vi "Simulation Record Get.vi"(8 "Error In":errorcluster, 11 "simulator":T20={"configuration"={"maxTime"=5.0, "enableVisualization"=TRUE, "Environment Definition"=path "iRobot Navigation State Machine.vi", "Record Location"=path "Simulation Record.xml", "autograde?"=TRUE, "interactive?"=FALSE, "Feedback Mode"=enum."debug navigation", "Robot State Charts"=[path "C:/Users/blueuser/Desktop/Robo Sim Berkley/cpsgrader-release-0.4/Simulators/EECS149lab/src/LabVIEW/statechart/Simulation Statechart.vi"], "statechart"=path "C:/Users/blueuser/Desktop/Robo Sim Berkley/cpsgrader-release-0.4/Simulators/EECS149lab/src/LabVIEW/statechart/Simulation Statechart.vi"}, "Statechart\ndisplay"=refnum, "first step?"=FALSE, "Robots Simulation Statecharts"=[], "Robots"=[]}) -> (0 "Error Out":errorcluster, 2 "record":T1={"configuration"={"maxTime"=5.0, "enableVisualization"=TRUE, "Environment Definition"=path "iRobot Navigation State Machine.vi", "Record Location"=path "Simulation Record.xml", "autograde?"=TRUE, "interactive?"=FALSE, "Feedback Mode"=enum."debug navigation", "Robot State Charts"=[path "C:/Users/blueuser/Desktop/Robo Sim Berkley/cpsgrader-release-0.4/Simulators/EECS149lab/src/LabVIEW/statechart/Simulation Statechart.vi"], "statechart"=path "C:/Users/blueuser/Desktop/Robo Sim Berkley/cpsgrader-release-0.4/Simulators/EECS149lab/src/LabVIEW/statechart/Simulation Statechart.vi"}, "trace"=[], "environment MD5"="", "statechart MD5"="", "record timestamp"=""} {"trace"."sensors"."Kobuki Sensors"."Infrared" format="%02x"; "trace"."sensors"."iRobot Sensors"."Infrared" format="%02x"; "trace"."sensors"."accelerometer"."z axis (g)" format="%.3f"; "trace"."sensors"."accelerometer"."y axis (g)" format="%.3f"; "trace"."sensors"."accelerometer"."x axis (g)" format="%.3f"}, 3 "simulator":T20={"configuration"={"maxTime"=5.0, "enableVisualization"=TRUE, "Environment Definition"=path "iRobot Navigation State Machine.vi", "Record Location"=path "Simulation Record.xml", "autograde?"=TRUE, "interactive?"=FALSE, "Feedback Mode"=enum."debug navigation", "Robot State Charts"=[path "C:/Users/blueuser/Desktop/Robo Sim Berkley/cpsgrader-release-0.4/Simulators/EECS149lab/src/LabVIEW/statechart/Simulation Statechart.vi"], "statechart"=path "C:/Users/blueuser/Desktop/Robo Sim Berkley/cpsgrader-release-0.4/Simulators/EECS149lab/src/LabVIEW/statechart/Simulation Statechart.vi"}, "Statechart\ndisplay"=refnum, "first step?"=FALSE, "Robots Simulation Statecharts"=[], "Robots"=[]})   [LabVIEW 2014]
uses:
  Simulator.ctl
  CyberSim interface/Simulation Configuration.ctl
  autograder/feedbackMode.ctl
  Multi Bot Code/RobotData.ctl
  <instrlib>/DC Motor Controller/HAIOL/DC Motor Controller.lvclass
  Simulation Record.ctl
  Simulation Trace Element.ctl
  shared/Sensors.ctl
  iRobot/Sensor/Accelerometer.ctl
  iRobot/Sensor/Sensor Group 6.ctl
  iRobot/Sensor/Bumps + Wheel Drops.ctl
  iRobot/Sensor/Buttons.ctl
  iRobot/Sensor/Charging State.ctl
  iRobot/Sensor/Charging Sources Available.ctl
  iRobot/Sensor/OI Mode.ctl
  iRobot/Sensor/Cargo Bay Digital Inputs.ctl
  iRobot/Sensor/Low-Side Driver + Wheel Overcurrent.ctl
  Kobuki/KobukiSensors.ctl
  Kobuki/Kobuki Bumps and WheelDrops.ctl
  Kobuki/Kobuki Buttons.ctl
  Simulated iRobot Position.ctl
  Simulated iRobot Orientation.ctl
  Simulation Trace Operation.ctl
panel:
  # "Electrical: charging, battery, OI mode"
  # "Sensors: bump, cliff, button, wheel drop, wall, virtual wall"
  # "Motors:"
  # "Cargo Bay: I/O, overcurrent, infrared"
  # "Song"
  # "Inertia"
  # "Electrical: charging, battery, OI mode"
  # "Sensors: bump, cliff, button, wheel drop, wall, virtual wall"
  # "Motion: distance, angle, requested velocity"
  # "Cargo Bay: I/O, overcurrent, infrared"
  # "Song"
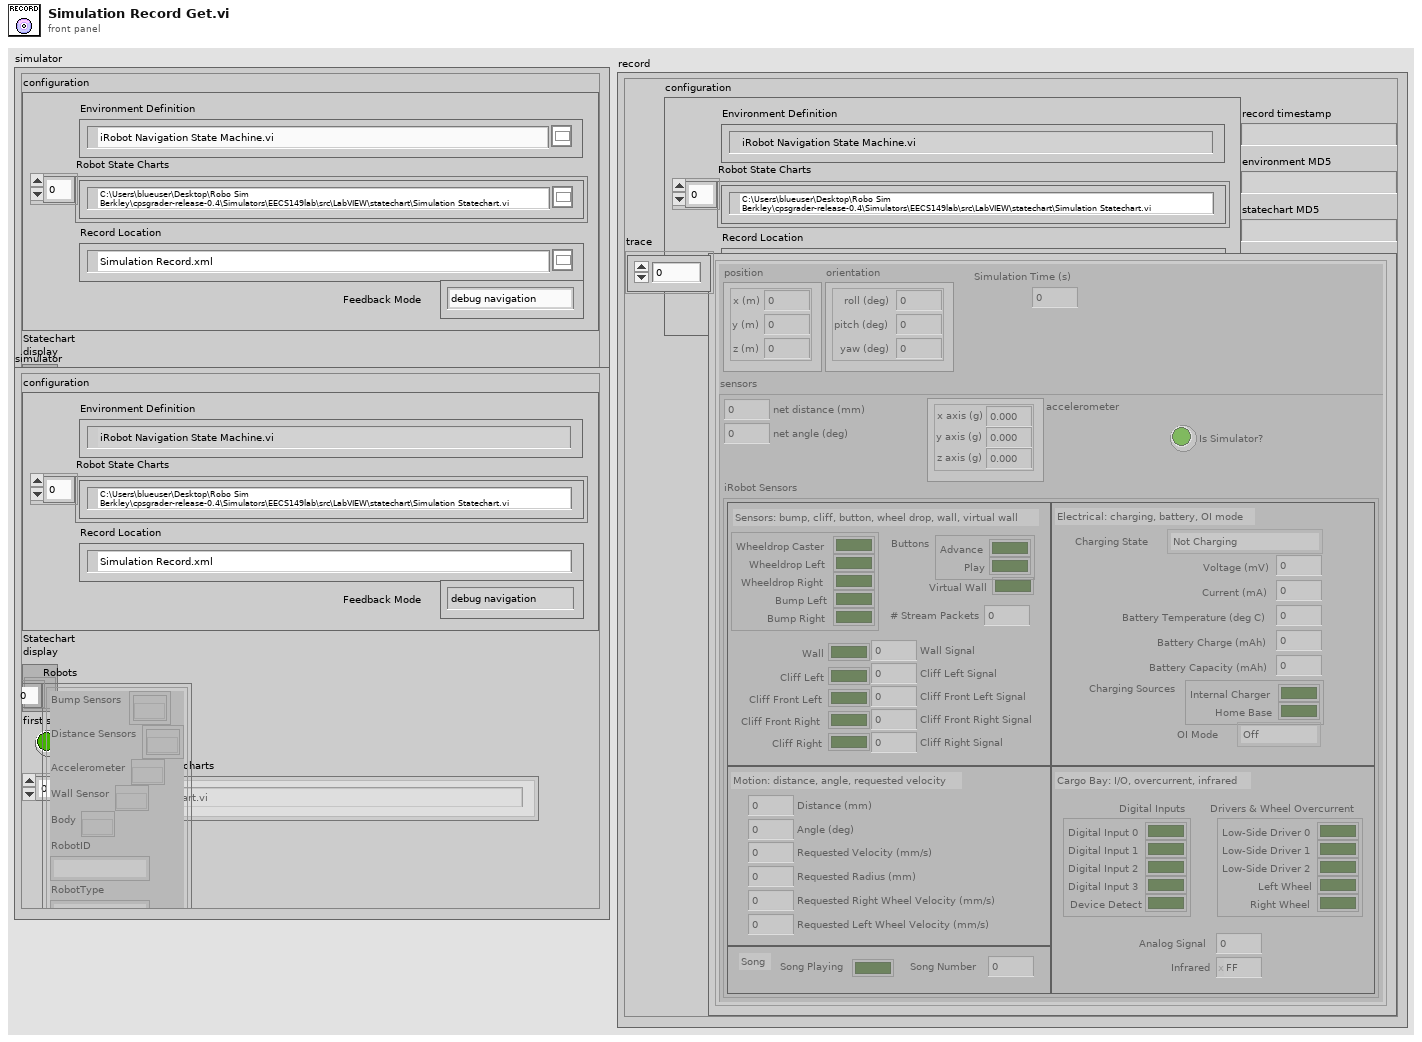
[diagram p1: front panel]
types:
  T1 = typedef "Simulation Record.ctl" = cluster{"configuration":T2, "trace":T4[], "environment MD5":string, "statechart MD5":string, "record timestamp":string}
  T2 = typedef "Simulation Configuration.ctl" = cluster{"maxTime":sgl, "enableVisualization":bool, "Environment Definition":path, "Record Location":path, "autograde?":bool, "interactive?":bool, "Feedback Mode":T3, "Robot State Charts":path[], "statechart":path}
  T3 = typedef "feedbackMode.ctl" = enum32{"debug navigation", "debug hill climb", "autograde navigation", "autograde hill climb"}
  T4 = typedef "Simulation Trace Element.ctl" = cluster{"sensors":T5, "position":T18, "orientation":T19, "Simulation Time (s)":sgl}
  T5 = typedef "Sensors.ctl" = cluster{"net distance (mm)":i32, "net angle (deg)":i32, "accelerometer":T6, "iRobot Sensors":T7, "Is Simulator?":bool, "Kobuki Sensors":T15}
  T6 = typedef "Accelerometer.ctl" = cluster{"x axis (g)":dbl, "y axis (g)":dbl, "z axis (g)":dbl}
  T7 = typedef "Sensor Group 6.ctl" = cluster{"Bumps + Wheel Drops":T8, "Wall":bool, "Cliff Left":bool, "Cliff Front Left":bool, "Cliff Front Right":bool, "Cliff Right":bool, "Wall Signal":u16, "Cliff Left Signal":u16, "Cliff Front Left Signal":u16, "Cliff Front Right Signal":u16, "Cliff Right Signal":u16, "Buttons":T9, "Virtual Wall":bool, "# Stream Packets":u8, "Requested Velocity (mm/s)":i16, "Requested Radius (mm)":i16, "Requested Right Wheel Velocity (mm/s)":i16, "Requested Left Wheel Velocity (mm/s)":i16, "Distance (mm)":i32, "Angle (deg)":i32, "Song Playing":bool, "Song Number":u8, "Charging State":T10, "Voltage (mV)":u16, "Current (mA)":i16, "Battery Temperature (deg C)":i8, "Battery Charge (mAh)":u16, "Battery Capacity (mAh)":u16, "Charging Sources":T11, "OI Mode":T12, "Digital Inputs":T13, "Drivers & Wheel Overcurrent":T14, "Analog Signal":u16, "Infrared":u8}
  T8 = typedef "Bumps + Wheel Drops.ctl" = cluster{"Wheeldrop Caster":bool, "Wheeldrop Left":bool, "Wheeldrop Right":bool, "Bump Left":bool, "Bump Right":bool}
  T9 = typedef "Buttons.ctl" = cluster{"Advance":bool, "Play":bool}
  T10 = typedef "Charging State.ctl" = enum16{"Not Charging", "Reconditioning Charging", "Full Charging", "Trickle Charging", "Waiting", "Charging Fault Condition"}
  T11 = typedef "Charging Sources Available.ctl" = cluster{"Internal Charger":bool, "Home Base":bool}
  T12 = typedef "OI Mode.ctl" = enum16{"Off", "Passive", "Safe", "Full"}
  T13 = typedef "Cargo Bay Digital Inputs.ctl" = cluster{"Digital Input 0":bool, "Digital Input 1":bool, "Digital Input 2":bool, "Digital Input 3":bool, "Device Detect":bool}
  T14 = typedef "Low-Side Driver + Wheel Overcurrent.ctl" = cluster{"Low-Side Driver 0":bool, "Low-Side Driver 1":bool, "Low-Side Driver 2":bool, "Left Wheel":bool, "Right Wheel":bool}
  T15 = typedef "KobukiSensors.ctl" = cluster{"Bumps + Wheel Drops":T16, "Cliff Left":bool, "Cliff Center":bool, "Cliff Right":bool, "Cliff Left Signal":i16, "Cliff Center Signal":i16, "Cliff Right Signal":i16, "Buttons":T17, "Left Wheel Encoder (ticks)":i16, "Song Playing":bool, "Song Number":u8, "Charging State":T10, "Voltage (mV)":i16, "Current (mA)":i16, "Battery Temperature (deg C)":i16, "Battery Charge (mAh)":i16, "Battery Capacity (mAh)":i16, "Charging Sources":T11, "OI Mode":T12, "Digital Inputs":T13, "Drivers & Wheel Overcurrent":T14, "Infrared":u8, "Right Wheel Encoder (ticks) ":i16, "TimeStamp":u16, "Right Wheel Current (x10mA)":i16, "Left  Wheel Current  (x10mA)":i16, "Angle( of 100deg)":i16, "Angle Rate( of 100 deg/sec)":i16}
  T16 = typedef "Kobuki Bumps and WheelDrops.ctl" = cluster{"Wheeldrop Left":bool, "Wheeldrop Right":bool, "Bump Left":bool, "Bump Center":bool, "Bump Right":bool}
  T17 = typedef "Kobuki Buttons.ctl" = cluster{"B0":bool, "B1":bool, "B2":bool}
  T18 = typedef "Simulated iRobot Position.ctl" = cluster{"x (m)":sgl, "y (m)":sgl, "z (m)":sgl}
  T19 = typedef "Simulated iRobot Orientation.ctl" = cluster{"roll (deg)":sgl, "pitch (deg)":sgl, "yaw (deg)":sgl}
  T20 = typedef "Simulator.ctl" = cluster{"configuration":T2, "Statechart\ndisplay":refnum<vi>, "first step?":bool, "Robots Simulation Statecharts":path[], "Robots":T21[]}
  T21 = typedef "RobotData.ctl" = cluster{"Bump Sensors":refnum<k20>[], "Distance Sensors":refnum<k20>[], "Accelerometer":refnum<k20>, "Wall Sensor":refnum<k20>, "Body":refnum<k20>, "RobotID":string, "RobotType":string, "Left Motor":refnum<class "DC Motor Controller.lvclass">, "Right Motor":refnum<class "DC Motor Controller.lvclass">}
  T22 = typedef "Simulation Trace Operation.ctl" = enum16{"Initialize", "Record Trace Element", "Get Trace"}
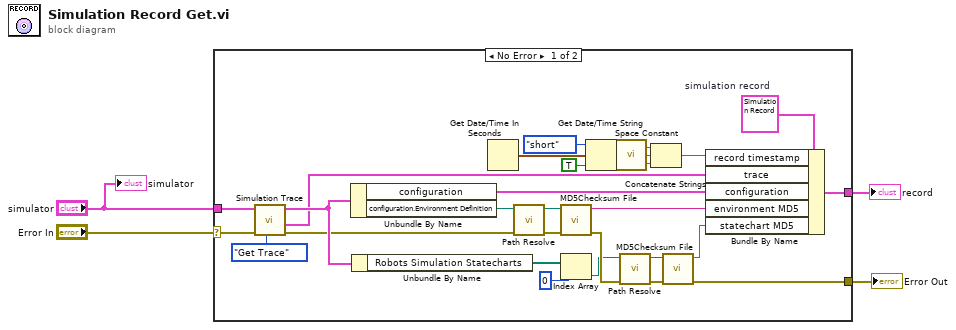
[diagram p0: block diagram]
diagram:
  n1 = case shown="No Error" "Error In" {
    selector: "Error In" -> [w8 w33]
    tunnel: [w32 w33] -> w4
    tunnel: "simulator" -> [w31 _]
    tunnel: [w30 _] -> w3
    frame No Error {
      w28 = T1 {"configuration"={"maxTime"=0.0, "enableVisualization"=FALSE, "Environment Definition"=path "", "Record Location"=path "", "autograde?"=FALSE, "interactive?"=FALSE, "Feedback Mode"=enum."debug navigation", "Robot State Charts"=[path "C:/Users/blueuser/Desktop/Robo Sim Berkley/cpsgrader-release-0.4/Simulators/EECS149lab/src/LabVIEW/statechart/Simulation Statechart.vi"], "statechart"=path "C:/Users/blueuser/Desktop/Robo Sim Berkley/cpsgrader-release-0.4/Simulators/EECS149lab/src/LabVIEW/statechart/Simulation Statechart.vi"}, "trace"=[], "environment MD5"="", "statechart MD5"="", "record timestamp"=""}  # simulation record
      n2 = call "Simulation Trace.vi"("operation"=Simulation_Trace_Operation."Get Trace", "error in"=w8, "simulator"=w31) -> ("error out"=w19:errorcluster, "trace"=w23:T4[], "simulator"=w29:T20)  [unwired: 5 in, 1 out]
      n3 = Unbundle By Name(w29) -> ("configuration"=w25:T2, "configuration.Environment Definition"=w20:path)
      n4 = Unbundle By Name(w29) -> ("Robots Simulation Statecharts"=w7:path[])
      n5 = Get Date/Time In Seconds() -> (seconds since 1Jan1904=w10:timestamp)
      n6 = call "Path Resolve.vi"("Error In"=w19, "absolute or relative path"=w20) -> ("Error Out"=w22:errorcluster, "resolved path"=w21:path)  [unwired: 8 in]
      n7 = call <vilib>:"MD5Checksum File.vi"("error in (no error)"=w22, "Path"=w21) -> ("error out"=w16:errorcluster, "MD5 message-digest"=w27:string)  [unwired: 8 in]
      n8 = Index Array(array=w7, index=0) -> (element=w5:path)
      n9 = Get Date/Time String(date format (0)=enum16{"short", "long", "abbreviated"}."short", seconds (now)=w10, want seconds? (F)=TRUE) -> (date string=w13:string, time string=w12:string)
      n10 = call <vilib>:"Space Constant.vi"() -> ("String"=w11:string)
      n11 = call "Path Resolve.vi"("Error In"=w16, "absolute or relative path"=w5) -> ("Error Out"=w17:errorcluster, "resolved path"=w18:path)  [unwired: 8 in]
      n12 = Concatenate Strings(w13, w11, w12) -> (w9:string)
      n13 = call <vilib>:"MD5Checksum File.vi"("error in (no error)"=w17, "Path"=w18) -> ("error out"=w32:errorcluster, "MD5 message-digest"=w26:string)  [unwired: 8 in]
      n14 = Bundle By Name(cluster=w28, "record timestamp"=w9, "trace"=w23, "configuration"=w25, "environment MD5"=w27, "statechart MD5"=w26) -> (w30:T1)
    }
    frame Error {
    }
  }
  "Error Out" <- w4
  "record" <- w3
  "simulator" <- "simulator"
